vi "Construct.vi"(0 "Commit Behavior Config File":path, 1 "Component Root Path":path, 11 "error in (no error)":errorcluster) -> (4 "Commit out":refnum<class "Commit.lvclass">, 15 "error out":errorcluster)   [LabVIEW 2017, in "CL_G3_VIComponentBuilder.lvlib" / "Commit.lvclass"]
doc: "Brings the Commit object into existence and sets the initial values according to the Commit Behavior Config File."
uses:
  Commit.lvclass
  Commit.lvclass/Commit.ctl
  Accessors/Write Commit Config File.vi
  Accessors/Write Component Root Path.vi
  <vilib>/Utility/libraryn.llb/Check if File or Folder Exists.vi
  <vilib>/Utility/error.llb/Error Cluster From Error Code.vi
  <vilib>/Utility/config.llb/NI_LVConfig.lvlib
  CL_G3_VIComponentBuilder.lvlib
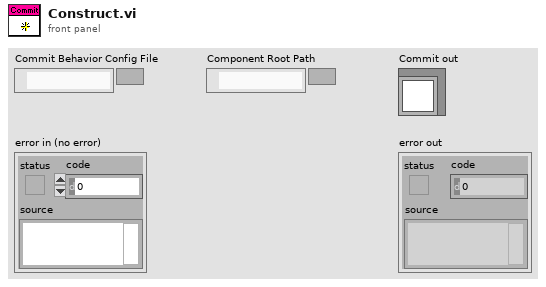
[diagram p1: front panel]
types:
  T1 = typedef "NI_LVConfig.lvlib/Config Data RefNum.ctl" = refnum<k1>
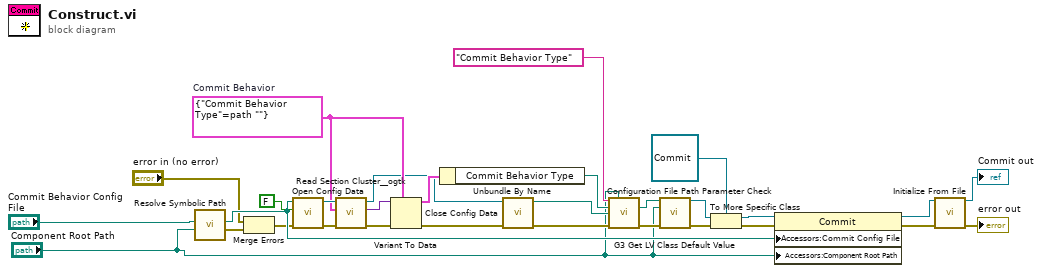
[diagram p0: block diagram]
diagram:
  w18 = cluster{"Commit Behavior Type":path} {"Commit Behavior Type"=path ""}  # Commit Behavior
  n1 = call "Resolve Symbolic Path.vi"("Component Root Path"="Component Root Path", "Path In"="Commit Behavior Config File") -> ("error out"=w3:errorcluster, "Path Out"=w11:path)  [unwired: 8 in]
  n2 = Merge Errors("error in (no error)", w3) -> (w2:errorcluster)
  n3 = call <vilib>:"Open Config Data.vi"("error in (no error)"=w2, "create file if necessary (T)"=FALSE, "configuration file path"=w11) -> ("error out"=w22:errorcluster, "refnum"=w24:T1)  [unwired: 6 in, 1 out]
  n4 = call <userlib>:"Read Section Cluster__ogtk.vi"("error in (no error)"=w22, "Section Formatted Cluster Type"=w18, "refnum"=w24) -> ("error out"=w21:errorcluster, "Section Formatted Cluster"=w23:variant, "dup refnum"=w17:T1)  [unwired: 4 in, 2 out]
  n5 = Variant To Data(error in=w21, type=w18, Variant=w23) -> (data=w20:cluster{"Commit Behavior Type":path}, error out=w16:errorcluster)
  n6 = Unbundle By Name(w20) -> ("Commit Behavior Type"=w9:path)
  n7 = call <vilib>:"Close Config Data.vi"("error in (no error)"=w16, "refnum"=w17) -> ("error out"=w6:errorcluster, "file path"=w8:path)  [unwired: 8 in]
  n8 = call "Configuration File Path Parameter Check.vi"("Parameter Name"="Commit Behavior Type", "Component Root Path"="Component Root Path", "Specified Path in Configuration File"=w9, "Configuration File Path"=w8, "error in (no error)"=w6) -> ("dup Specified Path in Configuration File"=w7:path, "error out"=w5:errorcluster)  [unwired: 8 in, 1 out]
  n9 = call "G3 Get LV Class Default Value.vi"("Export Type"=w7, "Component Definition ini Path"="Component Root Path", "error in (no error)"=w5) -> ("LabVIEW Object out"=w30:refnum<class>, "error out"=w19:errorcluster)  [unwired: 11 in]
  n10 = To More Specific Class(target class=refnum<class "Commit.lvclass"> refnum ("Commit"), reference=w30, error in=w19) -> (specific class reference=w28:refnum<class "Commit.lvclass">, error out=w14:errorcluster)
  n11 = property class="Commit"(reference=w28, error in=w14, "Accessors:Commit Config File"=w11, "Accessors:Component Root Path"="Component Root Path") -> (reference out=w15:refnum<class "Commit.lvclass">, error out=w13:errorcluster)
  n12 = call-dynamic "Initialize From File.vi"("Commit in"=w15, "error in (no error)"=w13) -> ("Commit out"=→"Commit out":refnum<class "Commit.lvclass">, "error out"=→"error out":errorcluster)  [unwired: 12 in]
